vi "Restart ADB Server.vi"(0 "adb location":string, 1 "error in":errorcluster) -> (4 "error out":errorcluster)   [LabVIEW 2016]
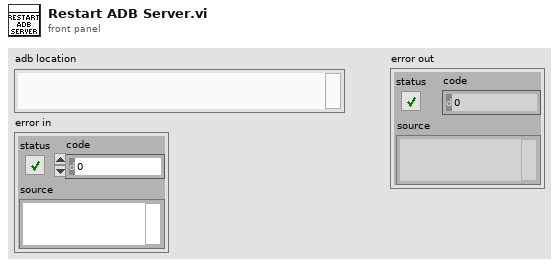
[diagram p1: front panel]
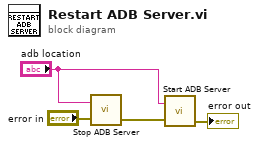
[diagram p0: block diagram]
diagram:
  n1 = call "Stop ADB Server.vi"("adb location"="adb location", "error in"="error in") -> ("error out"=w1:errorcluster)  [unwired: 2 out]
  n2 = call "Start ADB Server.vi"("adb location"="adb location", "error in"=w1) -> ("error out"=→"error out":errorcluster)  [unwired: 2 in]
